vi "Conjugate Gradient nD.vi"(4 "f(X)":string, 5 "accuracy":dbl=1e-08 format="%.2e", 6 "X":string[](array[string]), 7 "Start":dbl[](array[numeric]) format="%.2f", 8 "line minimization":u16(ring) items=["without derivatives", "with derivatives"], 9 "gradient method":u16(ring) items=["Fletcher-Reeves", "Polak-Ribiere"]) -> (0 "error":i32, 1 "ticks":u32, 2 "f(Minimum)":dbl format="%.2f", 3 "Minimum":dbl[](array[numeric]) format="%.2f")   [LabVIEW 2017, in "NI_Gmath.lvlib"]
doc: "Determines a local minimum of a function of n independent variables with the Conjugate Gradient method."
uses:
  NI_Gmath.lvlib
  Real Dot Product.vi
  NI_AALBase.lvlib
panel:
  # "Example:\n\n accuracy: 1E-8 \n gradient method: Fletcher-Reeves \n line minimization: without derivatives \n Start: 0.0 and 0.0 \n X: x and y\n f(X): x^2+y^2+sin(x-y)"
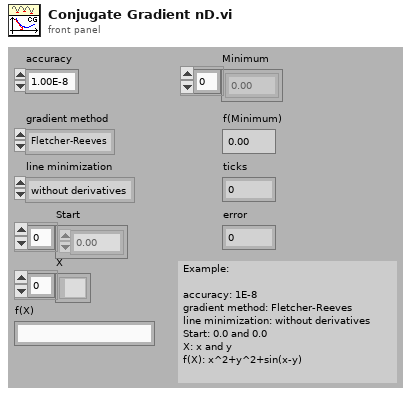
[diagram p1: front panel]
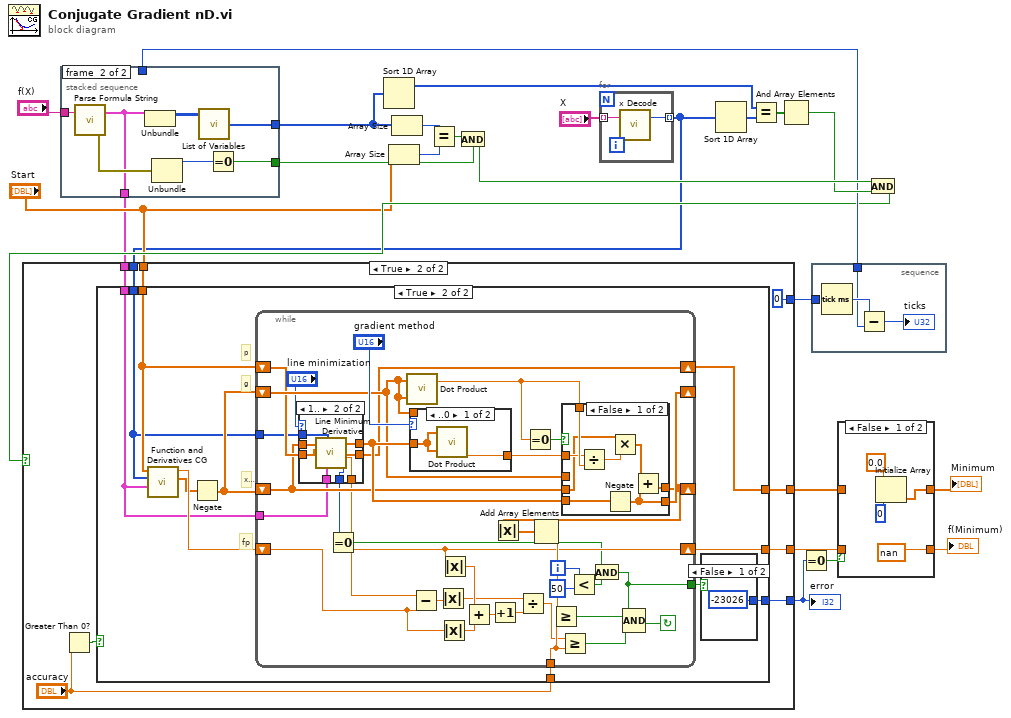
[diagram p0: block diagram]
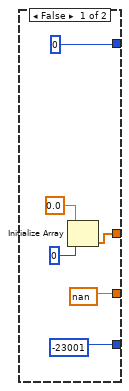
[diagram p3: hidden frame]
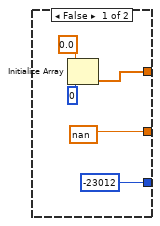
[diagram p4: hidden frame]
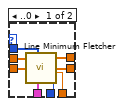
[diagram p5: hidden frame]
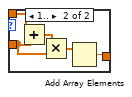
[diagram p6: hidden frame]
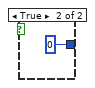
[diagram p8: hidden frame]
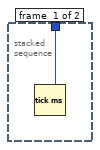
[diagram p9: hidden frame]
diagram:
  n1 = stacked-sequence {
    tunnel: [_ w32] -> w14
    tunnel: [w25 _] -> w13
    tunnel: [_ w31] -> w24
    tunnel: "f(X)" -> [_ w30]
    tunnel: [_ w26] -> w2
    frame #0 {
      n2 = Tick Count (ms)() -> (millisecond timer value=w25:u32)
    }
    frame #1 {
      n3 = call "Parse Formula String.vi"("formula"=w30) -> ("error out"=w29:errorcluster, "Parsed Formula"=w26:cluster{"Table":i32[][], "Y Values":dbl[]})  [unwired: 1 in]
      n4 = Unbundle(w26) -> ("Table"=w27:i32[][])  [unwired: 1 out]
      n5 = Unbundle(w29) -> ("code"=w28:i32)  [unwired: 2 out]
      n6 = call "List of Variables.vi"("Table"=w27) -> ("List of variables"=w31:i32[])
      n7 = Equal To 0?(x=w28) -> (x = 0?=w32:bool)
    }
  }
  n8 = Sort 1D Array(array=w24) -> (sorted array=w21:i32[])
  n9 = Array Size(array="Start") -> (size(s)=w22:i32)
  n10 = Array Size(array=w24) -> (size(s)=w23:i32)
  n11 = Equal?(x=w22, y=w23) -> (x = y?=w18:bool)
  n12 = And(x=w18, y=w14) -> (x .and. y?=w17:bool)
  n13 = for {
    tunnel: "X" -> [w34] mode=indexing
    tunnel: [w33] -> w1 mode=indexing
    n14 = call "x Decode.vi"("x string"=w34) -> ("number"=w33:i32)  [unwired: 1 in, 1 out]
  }
  n15 = Sort 1D Array(array=w1) -> (sorted array=w20:i32[])
  n16 = Equal?(x=w21, y=w20) -> (x = y?=w19:bool[])
  n17 = And Array Elements(Boolean array=w19) -> (logical AND=w16:bool)
  n18 = And(x=w17, y=w16) -> (x .and. y?=w11:bool)
  n19 = case shown="True" w11 {
    tunnel: "Start" -> [_ w49]
    tunnel: [0 0] -> w12
    tunnel: [nan w47] -> w5
    tunnel: [w37 w43] -> w7
    tunnel: [-23001 w44] -> w9
    tunnel: w2 -> [_ w42]
    tunnel: w1 -> [_ w41]
    frame False {
      n20 = Initialize Array(0.0, 0) -> (w37:dbl[])
    }
    frame True {
      n21 = Greater Than 0?(x="accuracy") -> (x > 0?=w45:bool)
      n22 = case shown="True" w45 {
        tunnel: [w52 w57] -> w43
        tunnel: [nan w65] -> w47
        tunnel: "accuracy" -> [_ w64]
        tunnel: w49 -> [_ w60]
        tunnel: [-23012 w58] -> w44
        tunnel: w42 -> [_ w56]
        tunnel: w41 -> [_ w55]
        frame False {
          n23 = Initialize Array(0.0, 0) -> (w52:dbl[])
        }
        frame True {
          # "fp"
          # "xi"
          # "g"
          # "p"
          n24 = call "Function and Derivatives CG.vi"("Parsed Formula"=w56, "Variables"=w55, "X"=w60) -> ("df/dX"=w62:dbl[], "f(X)"=w63:dbl)  [unwired: 7 in]
          n25 = Negate(x=w62) -> (-x=w61:dbl[])
          n26 = while {
            tunnel: [w68] -> w59
            tunnel: w64 -> [w81]
            shift-left: w63 -> [w97]
            shift-right: [w72] -> w65
            shift-left: w61 -> [w74]
            shift-right: [w73] -> _
            shift-left: w61 -> [w87]
            shift-right: [w98] -> _
            shift-left: w60 -> [w75]
            shift-right: [w78] -> w57
            tunnel: w56 -> [w67]
            tunnel: w55 -> [w66]
            i -> [w84]
            stop <- w79 continue-if-true
            n27 = case shown="1.." "line minimization" {
              tunnel: [w108 w116] -> w89
              tunnel: [w104 w112] -> w72
              tunnel: [w105 w115] -> w78
              tunnel: w74 -> [w107 w114]
              tunnel: w75 -> [w106 w113]
              tunnel: [w103 w111] -> w71
              tunnel: w67 -> [w102 w109]
              tunnel: w66 -> [w101 w110]
              frame ..0 {
                n28 = call "Line Minimum Fletcher.vi"("Parsed Formula"=w102, "Variables"=w101, "p"=w106, "xit"=w107) -> ("error"=w103:i32, "f(p)"=w104:dbl, "pnew"=w105:dbl[], "xitnew"=w108:dbl[])  [unwired: 4 in]
              }
              frame 1.. {
                n29 = call "Line Minimum Derivative.vi"("Parsed Formula"=w109, "Variables"=w110, "p"=w113, "xit"=w114) -> ("error"=w111:i32, "f(p)"=w112:dbl, "pnew"=w115:dbl[], "xitnew"=w116:dbl[])  [unwired: 4 in]
              }
            }
            n30 = Equal To 0?(x=w71) -> (x = 0?=w70:bool)
            n31 = call-poly "Dot Product.vi"("Y Vector"=w87, "X Vector"=w87) -> ("X * Y"=w90:dbl)  [unwired: 1 out]
            n32 = case shown="..0" "gradient method" {
              tunnel: w89 -> [w118 w121]
              tunnel: [w117 w119] -> w99
              tunnel: w87 -> [_ w123]
              frame ..0 {
                n33 = call-poly "Dot Product.vi"("Y Vector"=w118, "X Vector"=w118) -> ("X * Y"=w117:dbl)  [unwired: 1 out]
              }
              frame 1.. {
                n34 = Add(x=w123, y=w121) -> (x+y=w122:dbl[])
                n35 = Multiply(x=w122, y=w121) -> (x*y=w120:dbl[])
                n36 = Add Array Elements(numeric array=w120) -> (sum=w119:dbl)
              }
            }
            n37 = Subtract(x=w72, y=w97) -> (x-y=w96:dbl)
            n38 = Absolute Value(x=w96) -> (abs(x)=w93:dbl)
            n39 = Absolute Value(x=w97) -> (abs(x)=w94:dbl)
            n40 = Absolute Value(x=w72) -> (abs(x)=w95:dbl)
            n41 = Add(x=w95, y=w94) -> (x+y=w92:dbl)
            n42 = Increment(x=w92) -> (x+1=w91:dbl)
            n43 = Divide(x=w93, y=w91) -> (x/y=w76:dbl)
            n44 = Equal To 0?(x=w90) -> (x = 0?=w100:bool)
            n45 = Greater Or Equal?(x=w76, y=w81) -> (x >= y?=w80:bool)
            n46 = case shown="False" w100 {
              tunnel: w90 -> [w131 _]
              tunnel: w99 -> [w130 _]
              tunnel: w74 -> [w128 w133]
              tunnel: w89 -> [w127 _]
              tunnel: [w126 w132] -> w98
              tunnel: [w124 w133] -> w73
              tunnel: w87 -> [_ w132]
              frame False {
                n47 = Divide(x=w130, y=w131) -> (x/y=w129:dbl)
                n48 = Negate(x=w127) -> (-x=w126:dbl[])
                n49 = Multiply(x=w128, y=w129) -> (x*y=w125:dbl[])
                n50 = Add(x=w125, y=w126) -> (x+y=w124:dbl[])
              }
              frame True {
              }
            }
            n51 = Absolute Value(x=w73) -> (abs(x)=w83:dbl[])
            n52 = Add Array Elements(numeric array=w83) -> (sum=w82:dbl)
            n53 = Greater Or Equal?(x=w82, y=w81) -> (x >= y?=w77:bool)
            n54 = Less?(x=w84, y=50) -> (x < y?=w69:bool)
            n55 = And(x=w70, y=w69) -> (x .and. y?=w68:bool)
            n56 = Compound Arithmetic op=AND(w68, w77, w80) -> (w79:bool)
          }
          n57 = case shown="False" w59 {
            tunnel: [-23026 0] -> w58
            frame False {
            }
            frame True {
            }
          }
        }
      }
    }
  }
  "error" <- w9
  n58 = Equal To 0?(x=w9) -> (x = 0?=w8:bool)
  n59 = stacked-sequence {
    tunnel: w13 -> [w137]
    tunnel: w12 -> [_]
    frame #0 {
      n60 = Tick Count (ms)() -> (millisecond timer value=w138:u32)
      n61 = Subtract(x=w138, y=w137) -> (x-y=→"ticks":u32)
    }
  }
  n62 = case shown="False" w8 {
    tunnel: w7 -> [_ w144]
    tunnel: [w140 w144] -> w6
    tunnel: w5 -> [_ w143]
    tunnel: [nan w143] -> w4
    frame False {
      n63 = Initialize Array(0.0, 0) -> (w140:dbl[])
    }
    frame True {
    }
  }
  "f(Minimum)" <- w4
  "Minimum" <- w6
